vi "example_02_convert.vi"() -> ()   [LabVIEW 2015, in "lv-unit-conversion.lvlib"] (continued)
"is_si_unit"=TRUE, "category"="derived", "base_unit"="m/m3", "conversion_reference"="DERIVED", "is_exact"=TRUE, "a"=0.0, "b"=1000000.0, "c"=1.0, "d"=0.0, "underlying_def"="", "description"=""}, {"symbol"="mi/gal[UK]", "name"="mile per UK gallon", "dimension"="1/L2", "is_si_unit"=TRUE, "category"="derived", "base_unit"="m/m3", "conversion_reference"="DERIVED", "is_exact"=TRUE, "a"=0.0, "b"=1609.344, "c"=0.00454609, "d"=0.0, "underlying_def"="", "description"=""}, {"symbol"="mi/gal[US]", "name"="mile per US gallon", "dimension"="1/L2", "is_si_unit"=TRUE, "category"="derived", "base_unit"="m/m3", "conversion_reference"="DERIVED", "is_exact"=TRUE, "a"=0.0, "b"=1609.344, "c"=0.003785411784, "d"=0.0, "underlying_def"="", "description"=""}, {"symbol"="1/bbl", "name"="per barrel", "dimension"="1/L3", "is_si_unit"=TRUE, "category"="derived", "base_unit"="1/m3", "conversion_reference"="DERIVED", "is_exact"=TRUE, "a"=0.0, "b"=1.0, "c"=0.158987294928, "d"=0.0, "underlying_def"="", "description"=""}, {"symbol"="1/ft3", "name"="per cubic foot", "dimension"="1/L3", "is_si_unit"=TRUE, "category"="derived", "base_unit"="1/m3", "conversion_reference"="DERIVED", "is_exact"=TRUE, "a"=0.0, "b"=1.0, "c"=0.028316846592, "d"=0.0, "underlying_def"="", "description"=""}, {"symbol"="1/gal[UK]", "name"="per UK gallon", "dimension"="1/L3", "is_si_unit"=TRUE, "category"="derived", "base_unit"="1/m3", "conversion_reference"="DERIVED", "is_exact"=TRUE, "a"=0.0, "b"=1.0, "c"=0.00454609, "d"=0.0, "underlying_def"="", "description"=""}, {"symbol"="1/gal[US]", "name"="per US gallon", "dimension"="1/L3", "is_si_unit"=TRUE, "category"="derived", "base_unit"="1/m3", "conversion_reference"="DERIVED", "is_exact"=TRUE, "a"=0.0, "b"=1.0, "c"=0.003785411784, "d"=0.0, "underlying_def"="", "description"=""}, {"symbol"="1/L", "name"="per litre", "dimension"="1/L3", "is_si_unit"=TRUE, "category"="derived", "base_unit"="1/m3", "conversion_reference"="DERIVED", "is_exact"=TRUE, "a"=0.0, "b"=1000.0, "c"=1.0, "d"=0.0, "underlying_def"="", "description"=""}, {"symbol"="1/m3", "name"="per cubic metre", "dimension"="1/L3", "is_si_unit"=TRUE, "category"="derived", "base_unit"="", "conversion_reference"="", "is_exact"=FALSE, "a"=0.0, "b"=0.0, "c"=0.0, "d"=0.0, "underlying_def"="", "description"=""}, {"symbol"="1/g", "name"="per gram", "dimension"="1/M", "is_si_unit"=TRUE, "category"="derived", "base_unit"="1/kg", "conversion_reference"="DERIVED", "is_exact"=TRUE, "a"=0.0, "b"=1000.0, "c"=1.0, "d"=0.0, "underlying_def"="", "description"=""}, {"symbol"="1/lbm", "name"="per pound", "dimension"="1/M", "is_si_unit"=TRUE, "category"="derived", "base_unit"="1/kg", "conversion_reference"="DERIVED", "is_exact"=TRUE, "a"=0.0, "b"=1.0, "c"=0.45359237, "d"=0.0, "underlying_def"="", "description"=""}, {"symbol"="1/kg", "name"="per kilogram", "dimension"="1/M", "is_si_unit"=TRUE, "category"="derived", "base_unit"="", "conversion_reference"="", "is_exact"=FALSE, "a"=0.0, "b"=0.0, "c"=0.0, "d"=0.0, "underlying_def"="", "description"=""}, {"symbol"="1/(kg.s)", "name"="per (kilogram per second)", "dimension"="1/MT", "is_si_unit"=TRUE, "category"="derived", "base_unit"="Bq/kg", "conversion_reference"="DERIVED", "is_exact"=TRUE, "a"=0.0, "b"=1.0, "c"=1.0, "d"=0.0, "underlying_def"="", "description"=""}, {"symbol"="pCi/g", "name"="picocurie per gram", "dimension"="1/MT", "is_si_unit"=TRUE, "category"="derived", "base_unit"="Bq/kg", "conversion_reference"="DERIVED", "is_exact"=TRUE, "a"=0.0, "b"=37.0, "c"=1.0, "d"=0.0, "underlying_def"="", "description"=""}, {"symbol"="Bq/kg", "name"="becquerel per kilogram", "dimension"="1/MT", "is_si_unit"=TRUE, "category"="derived", "base_unit"="", "conversion_reference"="", "is_exact"=FALSE, "a"=0.0, "b"=0.0, "c"=0.0, "d"=0.0, "underlying_def"="1/(kg.s)", "description"=""}, {"symbol"="Ci", "name"="curie", "dimension"="1/T", "is_si_unit"=TRUE, "category"="atom-allowed", "base_unit"="Bq", "conversion_reference"="NIST-SI", "is_exact"=TRUE, "a"=0.0, "b"=37000000000.0, "c"=1.0, "d"=0.0, "underlying_def"="3.7E10 Bq", "description"="The Curie (symbol Ci) is a non-SI unit of radioactivity, named after Marie and Pierre Curie. \n\t\t\t\tIt is defined as 3.7E10 decays per second. \n\t\t\t\tThe SI derived unit of radioactivity is the becquerel (Bq), which equates to one decay per second.\n\t\t\t"}, {"symbol"="Bd", "name"="baud", "dimension"="1/T", "is_si_unit"=TRUE, "category"="atom-allowed", "base_unit"="", "conversion_reference"="", "is_exact"=FALSE, "a"=0.0, "b"=0.0, "c"=0.0, "d"=0.0, "underlying_def"="1/s", "description"="The baud rate is the number of distinct symbols transmitted per second, that is, the number of times \n\t\t\t\tper second the signal carrying the communication varies in strength or frequency. \n\t\t\t\tIf the symbols transmitted have only two states (on or off) then the baud rate is the same as the \n\t\t\t\ttransmission rate in bits per second. \n\t\t\t\t(Adapted from Russ Rowlett's \"A Dictionary of Units of Measurement\" at http://www.unc.edu/~rowlett/units/)\n\t\t\t"}, {"symbol"="Bq", "name"="becquerel", "dimension"="1/T", "is_si_unit"=TRUE, "category"="atom-special", "base_unit"="", "conversion_reference"="", "is_exact"=FALSE, "a"=0.0, "b"=0.0, "c"=0.0, "d"=0.0, "underlying_def"="1/s", "description"="The activity of a radionuclide decaying at the rate of one spontaneous nuclear transition per second"}, {"symbol"="Hz", "name"="hertz", "dimension"="1/T", "is_si_unit"=TRUE, "category"="atom-special", "base_unit"="", "conversion_reference"="", "is_exact"=FALSE, "a"=0.0, "b"=0.0, "c"=0.0, "d"=0.0, "underlying_def"="1/s", "description"="The frequency of a periodic phenomenon of which the period is 1 second."}, {"symbol"="1/a", "name"="per julian-year", "dimension"="1/T", "is_si_unit"=TRUE, "category"="derived", "base_unit"="1/s", "conversion_reference"="DERIVED", "is_exact"=TRUE, "a"=0.0, "b"=1.0, "c"=31557600.0, "d"=0.0, "underlying_def"="", "description"=""}, {"symbol"="1/d", "name"="per day", "dimension"="1/T", "is_si_unit"=TRUE, "category"="derived", "base_unit"="1/s", "conversion_reference"="DERIVED", "is_exact"=TRUE, "a"=0.0, "b"=1.0, "c"=86400.0, "d"=0.0, "underlying_def"="", "description"=""}, {"symbol"="1/h", "name"="per hour", "dimension"="1/T", "is_si_unit"=TRUE, "category"="derived", "base_unit"="1/s", "conversion_reference"="DERIVED", "is_exact"=TRUE, "a"=0.0, "b"=1.0, "c"=3600.0, "d"=0.0, "underlying_def"="", "description"=""}, {"symbol"="1/min", "name"="per minute", "dimension"="1/T", "is_si_unit"=TRUE, "category"="derived", "base_unit"="1/s", "conversion_reference"="DERIVED", "is_exact"=TRUE, "a"=0.0, "b"=1.0, "c"=60.0, "d"=0.0, "underlying_def"="", "description"=""}, {"symbol"="1/ms", "name"="per millisecond", "dimension"="1/T", "is_si_unit"=TRUE, "category"="derived", "base_unit"="1/s", "conversion_reference"="DERIVED", "is_exact"=TRUE, "a"=0.0, "b"=1000.0, "c"=1.0, "d"=0.0, "underlying_def"="", "description"=""}, {"symbol"="1/us", "name"="per microsecond", "dimension"="1/T", "is_si_unit"=TRUE, "category"="derived", "base_unit"="1/s", "conversion_reference"="DERIVED", "is_exact"=TRUE, "a"=0.0, "b"=1000000.0, "c"=1.0, "d"=0.0, "underlying_def"="", "description"=""}, {"symbol"="1/wk", "name"="per week", "dimension"="1/T", "is_si_unit"=TRUE, "category"="derived", "base_unit"="1/s", "conversion_reference"="DERIVED", "is_exact"=TRUE, "a"=0.0, "b"=1.0, "c"=604800.0, "d"=0.0, "underlying_def"="", "description"=""}, {"symbol"="byte/s", "name"="byte per second", "dimension"="1/T", "is_si_unit"=TRUE, "category"="derived", "base_unit"="bit/s", "conversion_reference"="DERIVED", "is_exact"=TRUE, "a"=0.0, "b"=8.0, "c"=1.0, "d"=0.0, "underlying_def"="", "description"=""}, {"symbol"="1/s", "name"="per second", "dimension"="1/T", "is_si_unit"=TRUE, "category"="derived", "base_unit"="", "conversion_reference"="", "is_exact"=FALSE, "a"=0.0, "b"=0.0, "c"=0.0, "d"=0.0, "underlying_def"="", "description"=""}, {"symbol"="bit/s", "name"="bit per second", "dimension"="1/T", "is_si_unit"=TRUE, "category"="derived", "base_unit"="", "conversion_reference"="", "is_exact"=FALSE, "a"=0.0, "b"=0.0, "c"=0.0, "d"=0.0, "underlying_def"="1/s", "description"="A unit of transmission speed, equal to one bit per second."}, {"symbol"="m3/(s.m3)", "name"="cubic metre per time cubic metre", "dimension"="1/T", "is_si_unit"=TRUE, "category"="derived", "base_unit"="", "conversion_reference"="", "is_exact"=FALSE, "a"=0.0, "b"=0.0, "c"=0.0, "d"=0.0, "underlying_def"="1/s", "description"=""}, {"symbol"="bbl/(d.acre.ft)", "name"="barrel per day acre foot", "dimension"="1/T", "is_si_unit"=TRUE, "category"="derived", "base_unit"="m3/(s.m3)", "conversion_reference"="DERIVED", "is_exact"=TRUE, "a"=0.0, "b"=2464298.1427778574, "c"=1651882180608000.0, "d"=0.0, "underlying_def"="", "description"=""}, {"symbol"="GBq", "name"="gigabecquerel", "dimension"="1/T", "is_si_unit"=TRUE, "category"="prefixed", "base_unit"="Bq", "conversion_reference"="DERIVED", "is_exact"=TRUE, "a"=0.0, "b"=1000000000.0, "c"=1.0, "d"=0.0, "underlying_def"="", "description"=""}, {"symbol"="MBq", "name"="megabecquerel", "dimension"="1/T", "is_si_unit"=TRUE, "category"="prefixed", "base_unit"="Bq", "conversion_reference"="DERIVED", "is_exact"=TRUE, "a"=0.0, "b"=1000000.0, "c"=1.0, "d"=0.0, "underlying_def"="", "description"=""}, {"symbol"="mCi", "name"="thousandth of curie", "dimension"="1/T", "is_si_unit"=TRUE, "category"="prefixed", "base_unit"="Bq", "conversion_reference"="DERIVED", "is_exact"=TRUE, "a"=0.0, "b"=37000000.0, "c"=1.0, "d"=0.0, "underlying_def"="", "description"=""}, {"symbol"="nCi", "name"="nanocurie", "dimension"="1/T", "is_si_unit"=TRUE, "category"="prefixed", "base_unit"="Bq", "conversion_reference"="DERIVED", "is_exact"=TRUE, "a"=0.0, "b"=37.0, "c"=1.0, "d"=0.0, "underlying_def"="", "description"=""}, {"symbol"="pCi", "name"="picocurie", "dimension"="1/T", "is_si_unit"=TRUE, "category"="prefixed", "base_unit"="Bq", "conversion_reference"="DERIVED", "is_exact"=TRUE, "a"=0.0, "b"=0.037, "c"=1.0, "d"=0.0, "underlying_def"="", "description"=""}, {"symbol"="TBq", "name"="terabecquerel", "dimension"="1/T", "is_si_unit"=TRUE, "category"="prefixed", "base_unit"="Bq", "conversion_reference"="DERIVED", "is_exact"=TRUE, "a"=0.0, "b"=1000000000000.0, "c"=1.0, "d"=0.0, "underlying_def"="", "description"=""}, {"symbol"="uCi", "name"="millionth of curie", "dimension"="1/T", "is_si_unit"=TRUE, "category"="prefixed", "base_unit"="Bq", "conversion_reference"="DERIVED", "is_exact"=TRUE, "a"=0.0, "b"=37000.0, "c"=1.0, "d"=0.0, "underlying_def"="", "description"=""}, {"symbol"="cHz", "name"="centihertz", "dimension"="1/T", "is_si_unit"=TRUE, "category"="prefixed", "base_unit"="Hz", "conversion_reference"="DERIVED", "is_exact"=TRUE, "a"=0.0, "b"=0.01, "c"=1.0, "d"=0.0, "underlying_def"="", "description"=""}, {"symbol"="dHz", "name"="decihertz", "dimension"="1/T", "is_si_unit"=TRUE, "category"="prefixed", "base_unit"="Hz", "conversion_reference"="DERIVED", "is_exact"=TRUE, "a"=0.0, "b"=0.1, "c"=1.0, "d"=0.0, "underlying_def"="", "description"=""}, {"symbol"="EHz", "name"="exahertz", "dimension"="1/T", "is_si_unit"=TRUE, "category"="prefixed", "base_unit"="Hz", "conversion_reference"="DERIVED", "is_exact"=TRUE, "a"=0.0, "b"=1e+18, "c"=1.0, "d"=0.0, "underlying_def"="", "description"=""}, {"symbol"="fHz", "name"="femtohertz", "dimension"="1/T", "is_si_unit"=TRUE, "category"="prefixed", "base_unit"="Hz", "conversion_reference"="DERIVED", "is_exact"=TRUE, "a"=0.0, "b"=1e-15, "c"=1.0, "d"=0.0, "underlying_def"="", "description"=""}, {"symbol"="GHz", "name"="gigahertz", "dimension"="1/T", "is_si_unit"=TRUE, "category"="prefixed", "base_unit"="Hz", "conversion_reference"="DERIVED", "is_exact"=TRUE, "a"=0.0, "b"=1000000000.0, "c"=1.0, "d"=0.0, "underlying_def"="", "description"=""}, {"symbol"="kHz", "name"="kilohertz", "dimension"="1/T", "is_si_unit"=TRUE, "category"="prefixed", "base_unit"="Hz", "conversion_reference"="DERIVED", "is_exact"=TRUE, "a"=0.0, "b"=1000.0, "c"=1.0, "d"=0.0, "underlying_def"="", "description"=""}, {"symbol"="mHz", "name"="millihertz", "dimension"="1/T", "is_si_unit"=TRUE, "category"="prefixed", "base_unit"="Hz", "conversion_reference"="DERIVED", "is_exact"=TRUE, "a"=0.0, "b"=0.001, "c"=1.0, "d"=0.0, "underlying_def"="", "description"=""}, {"symbol"="MHz", "name"="megahertz", "dimension"="1/T", "is_si_unit"=TRUE, "category"="prefixed", "base_unit"="Hz", "conversion_reference"="DERIVED", "is_exact"=TRUE, "a"=0.0, "b"=1000000.0, "c"=1.0, "d"=0.0, "underlying_def"="", "description"=""}, {"symbol"="nHz", "name"="nanohertz", "dimension"="1/T", "is_si_unit"=TRUE, "category"="prefixed", "base_unit"="Hz", "conversion_reference"="DERIVED", "is_exact"=TRUE, "a"=0.0, "b"=1e-09, "c"=1.0, "d"=0.0, "underlying_def"="", "description"=""}, {"symbol"="pHz", "name"="picohertz", "dimension"="1/T", "is_si_unit"=TRUE, "category"="prefixed", "base_unit"="Hz", "conversion_reference"="DERIVED", "is_exact"=TRUE, "a"=0.0, "b"=1e-12, "c"=1.0, "d"=0.0, "underlying_def"="", "description"=""}, {"symbol"="THz", "name"="terahertz", "dimension"="1/T", "is_si_unit"=TRUE, "category"="prefixed", "base_unit"="Hz", "conversion_reference"="DERIVED", "is_exact"=TRUE, "a"=0.0, "b"=1000000000000.0, "c"=1.0, "d"=0.0, "underlying_def"="", "description"=""}, {"symbol"="uHz", "name"="microhertz", "dimension"="1/T", "is_si_unit"=TRUE, "category"="prefixed", "base_unit"="Hz", "conversion_reference"="DERIVED", "is_exact"=TRUE, "a"=0.0, "b"=1e-06, "c"=1.0, "d"=0.0, "underlying_def"="", "description"=""}, {"symbol"="rad", "name"="radian", "dimension"="A", "is_si_unit"=TRUE, "category"="atom-special", "base_unit"="", "conversion_reference"="", "is_exact"=FALSE, "a"=0.0, "b"=0.0, "c"=0.0, "d"=0.0, "underlying_def"="", "description"="The radian is the plane angle between two radii of a circle that cut of, on the circumference,an arc \n\t\t\t\tequal in length to the radius.\n\t\t\t"}, {"symbol"="ccgr", "name"="centesimal-second", "dimension"="A", "is_si_unit"=TRUE, "category"="atom", "base_unit"="rad", "conversion_reference"="EPSG", "is_exact"=TRUE, "a"=0.0, "b"=0.0, "c"=2000000.0, "d"=0.0, "underlying_def"="1/100 cgr", "description"="One hundredth of a centesimal-minute."}, {"symbol"="cgr", "name"="centesimal-minute", "dimension"="A", "is_si_unit"=TRUE, "category"="atom", "base_unit"="rad", "conversion_reference"="EPSG", "is_exact"=TRUE, "a"=0.0, "b"=0.0, "c"=20000.0, "d"=0.0, "underlying_def"="1/100 gon", "description"="One hundredth of a centesimal degree (also known as grad, grade or gon)"}, {"symbol"="dega", "name"="angular degree", "dimension"="A", "is_si_unit"=TRUE, "category"="atom-allowed", "base_unit"="rad", "conversion_reference"="NIST-SI", "is_exact"=TRUE, "a"=0.0, "b"=0.0, "c"=180.0, "d"=0.0, "underlying_def"="", "description"="1/360 of a full circle = PI /180 radians"}, {"symbol"="gon", "name"="gon", "dimension"="A", "is_si_unit"=TRUE, "category"="atom", "base_unit"="rad", "conversion_reference"="EPSG", "is_exact"=TRUE, "a"=0.0, "b"=0.0, "c"=200.0, "d"=0.0, "underlying_def"="360/400 dega", "description"="1/400 of a turn (full circle). Also known as gradian, grad, or grade."}, {"symbol"="mila", "name"="angular mil", "dimension"="A", "is_si_unit"=TRUE, "category"="atom", "base_unit"="rad", "conversion_reference"="EPSG", "is_exact"=TRUE, "a"=0.0, "b"=0.0, "c"=3200.0, "d"=0.0, "underlying_def"="360/6400 dega", "description"="Angle subtended by 1/6400 part of a circle."}, {"symbol"="mina", "name"="angular minute", "dimension"="A", "is_si_unit"=TRUE, "category"="atom-allowed", "base_unit"="rad", "conversion_reference"="NIST-SI", "is_exact"=TRUE, "a"=0.0, "b"=0.0, "c"=10800.0, "d"=0.0, "underlying_def"="1/60 dega", "description"="1/60 of an angular degree. ((pi/180) / 60) radians"}, {"symbol"="rev", "name"="revolution", "dimension"="A", "is_si_unit"=TRUE, "category"="atom", "base_unit"="rad", "conversion_reference"="DEFINITION", "is_exact"=TRUE, "a"=0.0, "b"=2.0, "c"=1.0, "d"=0.0, "underlying_def"="360 dega", "description"="One complete 360 degree rotational cycle."}, {"symbol"="seca", "name"="angular second", "dimension"="A", "is_si_unit"=TRUE, "category"="atom-allowed", "base_unit"="rad", "conversion_reference"="NIST-SI", "is_exact"=TRUE, "a"=0.0, "b"=0.0, "c"=648000.0, "d"=0.0, "underlying_def"="1/60 mina", "description"="1/60 of an angular minute. ((pi/180) / 3600) radians"}, {"symbol"="0.001 seca", "name"="angular millisecond", "dimension"="A", "is_si_unit"=TRUE, "category"="derived", "base_unit"="rad", "conversion_reference"="DERIVED", "is_exact"=TRUE, "a"=0.0, "b"=0.0, "c"=648000000.0, "d"=0.0, "underlying_def"="", "description"=""}, {"symbol"="krad", "name"="kiloradian", "dimension"="A", "is_si_unit"=TRUE, "category"="prefixed", "base_unit"="rad", "conversion_reference"="DERIVED", "is_exact"=TRUE, "a"=0.0, "b"=1000.0, "c"=1.0, "d"=0.0, "underlying_def"="", "description"=""}, {"symbol"="mrad", "name"="milliradian", "dimension"="A", "is_si_unit"=TRUE, "category"="prefixed", "base_unit"="rad", "conversion_reference"="DERIVED", "is_exact"=TRUE, "a"=0.0, "b"=0.001, "c"=1.0, "d"=0.0, "underlying_def"="", "description"=""}, {"symbol"="Mrad", "name"="megaradian", "dimension"="A", "is_si_unit"=TRUE, "category"="prefixed", "base_unit"="rad", "conversion_reference"="DERIVED", "is_exact"=TRUE, "a"=0.0, "b"=1000000.0, "c"=1.0, "d"=0.0, "underlying_def"="", "description"=""}, {"symbol"="urad", "name"="microradian", "dimension"="A", "is_si_unit"=TRUE, "category"="prefixed", "base_unit"="rad", "conversion_reference"="DERIVED", "is_exact"=TRUE, "a"=0.0, "b"=1e-06, "c"=1.0, "d"=0.0, "underlying_def"="", "description"=""}, {"symbol"="rad/m", "name"="radian per metre", "dimension"="A/L", "is_si_unit"=TRUE, "category"="derived", "base_unit"="", "conversion_reference"="", "is_exact"=FALSE, "a"=0.0, "b"=0.0, "c"=0.0, "d"=0.0, "underlying_def"="", "description"=""}, {"symbol"="0.01 dega/ft", "name"="angular degree per hundred foot", "dimension"="A/L", "is_si_unit"=TRUE, "category"="derived", "base_unit"="rad/m", "conversion_reference"="DERIVED", "is_exact"=TRUE, "a"=0.0, "b"=0.0, "c"=5486.4, "d"=0.0, "underlying_def"="", "description"=""}, {"symbol"="1/30 dega/ft", "name"="angular degree per thirty foot", "dimension"="A/L", "is_si_unit"=TRUE, "category"="derived", "base_unit"="rad/m", "conversion_reference"="DERIVED", "is_exact"=TRUE, "a"=0.0, "b"=0.0, "c"=1645.92, "d"=0.0, "underlying_def"="", "description"=""}, {"symbol"="1/30 dega/m", "name"="angular degree per thirty metre", "dimension"="A/L", "is_si_unit"=TRUE, "category"="derived", "base_unit"="rad/m", "conversion_reference"="DERIVED", "is_exact"=TRUE, "a"=0.0, "b"=0.0, "c"=5400.0, "d"=0.0, "underlying_def"="", "description"="((pi/180) / 30) radian per metre"}, {"symbol"="dega/ft", "name"="angular degree per foot", "dimension"="A/L", "is_si_unit"=TRUE, "category"="derived", "base_unit"="rad/m", "conversion_reference"="DERIVED", "is_exact"=TRUE, "a"=0.0, "b"=0.0, "c"=54.864, "d"=0.0, "underlying_def"="", "description"=""}, {"symbol"="dega/m", "name"="angular degree per metre", "dimension"="A/L", "is_si_unit"=TRUE, "category"="derived", "base_unit"="rad/m", "conversion_reference"="DERIVED", "is_exact"=TRUE, "a"=0.0, "b"=0.0, "c"=180.0, "d"=0.0, "underlying_def"="", "description"=""}, {"symbol"="rad/ft", "name"="radian per foot", "dimension"="A/L", "is_si_unit"=TRUE, "category"="derived", "base_unit"="rad/m", "conversion_reference"="DERIVED", "is_exact"=TRUE, "a"=0.0, "b"=1.0, "c"=0.3048, "d"=0.0, "underlying_def"="", "description"=""}, {"symbol"="rev/ft", "name"="revolution per foot", "dimension"="A/L", "is_si_unit"=TRUE, "category"="derived", "base_unit"="rad/m", "conversion_reference"="DERIVED", "is_exact"=TRUE, "a"=0.0, "b"=2.0, "c"=0.3048, "d"=0.0, "underlying_def"="", "description"=""}, {"symbol"="rev/m", "name"="revolution per metre", "dimension"="A/L", "is_si_unit"=TRUE, "category"="derived", "base_unit"="rad/m", "conversion_reference"="DERIVED", "is_exact"=TRUE, "a"=0.0, "b"=2.0, "c"=1.0, "d"=0.0, "underlying_def"="", "description"=""}, {"symbol"="rad/m3", "name"="radian per cubic metre", "dimension"="A/L3", "is_si_unit"=TRUE, "category"="derived", "base_unit"="", "conversion_reference"="", "is_exact"=FALSE, "a"=0.0, "b"=0.0, "c"=0.0, "d"=0.0, "underlying_def"="", "description"=""}, {"symbol"="rad/ft3", "name"="radian per cubic foot", "dimension"="A/L3", "is_si_unit"=TRUE, "category"="derived", "base_unit"="rad/m3", "conversion_reference"="DERIVED", "is_exact"=TRUE, "a"=0.0, "b"=1.0, "c"=0.028316846592, "d"=0.0, "underlying_def"="", "description"=""}, {"symbol"="rpm", "name"="revolution per minute", "dimension"="A/T", "is_si_unit"=TRUE, "category"="atom", "base_unit"="rad/s", "conversion_reference"="DERIVED", "is_exact"=TRUE, "a"=0.0, "b"=2.0, "c"=60.0, "d"=0.0, "underlying_def"="rev/min", "description"=""}, {"symbol"="rad/s", "name"="radian per second", "dimension"="A/T", "is_si_unit"=TRUE, "category"="derived", "base_unit"="", "conversion_reference"="", "is_exact"=FALSE, "a"=0.0, "b"=0.0, "c"=0.0, "d"=0.0, "underlying_def"="", "description"=""}, {"symbol"="dega/h", "name"="angular degree per hour", "dimension"="A/T", "is_si_unit"=TRUE, "category"="derived", "base_unit"="rad/s", "conversion_reference"="DERIVED", "is_exact"=TRUE, "a"=0.0, "b"=0.0, "c"=648000.0, "d"=0.0, "underlying_def"="", "description"="((pi/180) / 3600) radian per second"}, {"symbol"="dega/min", "name"="angular degree per minute", "dimension"="A/T", "is_si_unit"=TRUE, "category"="derived", "base_unit"="rad/s", "conversion_reference"="DERIVED", "is_exact"=TRUE, "a"=0.0, "b"=0.0, "c"=10800.0, "d"=0.0, "underlying_def"="", "description"="((pi/180) / 60) radian per second"}, {"symbol"="dega/s", "name"="angular degree per second", "dimension"="A/T", "is_si_unit"=TRUE, "category"="derived", "base_unit"="rad/s", "conversion_reference"="DERIVED", "is_exact"=TRUE, "a"=0.0, "b"=0.0, "c"=180.0, "d"=0.0, "underlying_def"="", "description"="(pi/180) radian per second"}, {"symbol"="rev/s", "name"="revolution per second", "dimension"="A/T", "is_si_unit"=TRUE, "category"="derived", "base_unit"="rad/s", "conversion_reference"="DERIVED", "is_exact"=TRUE, "a"=0.0, "b"=2.0, "c"=1.0, "d"=0.0, "underlying_def"="", "description"=""}, {"symbol"="rad/s2", "name"="radian per second squared", "dimension"="A/T2", "is_si_unit"=TRUE, "category"="derived", "base_unit"="", "conversion_reference"="", "is_exact"=FALSE, "a"=0.0, "b"=0.0, "c"=0.0, "d"=0.0, "underlying_def"="", "description"=""}, {"symbol"="rpm/s", "name"="(revolution per minute) per second", "dimension"="A/T2", "is_si_unit"=TRUE, "category"="derived", "base_unit"="rad/s2", "conversion_reference"="DERIVED", "is_exact"=TRUE, "a"=0.0, "b"=2.0, "c"=60.0, "d"=0.0, "underlying_def"="", "description"=""}, {"symbol"="deltaC", "name"="delta Celsius", "dimension"="D", "is_si_unit"=TRUE, "category"="atom-special", "base_unit"="deltaK", "conversion_reference"="NIST-SI", "is_exact"=TRUE, "a"=0.0, "b"=1.0, "c"=1.0, "d"=0.0, "underlying_def"="deltaK", "description"="Change in degree Celsius. \n\t\t\t\tThe degree Celsius and the kelvin are equal in size, so that the numerical value of a temperature \n\t\t\t\tdifference or temperature interval is the same when expressed in either degrees Celsius or in \n\t\t\t\tkelvins (because the offset cancels). \n\t\t\t\tFor temperature intervals rather than specific temperatures, 1 deltaF = 1 deltaR = 5/9 deltaC = 5/9 deltaK.\n\t\t\t"}, {"symbol"="deltaF", "name"="delta Fahrenheit", "dimension"="D", "is_si_unit"=TRUE, "category"="atom", "base_unit"="deltaK", "conversion_reference"="NIST-SI", "is_exact"=TRUE, "a"=0.0, "b"=5.0, "c"=9.0, "d"=0.0, "underlying_def"="", "description"="Change in degrees Fahrenheit. \n\t\t\t\tKelvin=(Fahrenheit + 459.67) x 5/9 so a difference in Fahrenheit temperature cancels out the 459.67 \n\t\t\t\toffset. \n\t\t\t\tFor temperature intervals rather than specific temperatures, 1 deltaF = 1 deltaR = 5/9 deltaC = 5/9 deltaK.\n\t\t\t"}, {"symbol"="deltaR", "name"="delta Rankine", "dimension"="D", "is_si_unit"=TRUE, "category"="atom", "base_unit"="deltaK", "conversion_reference"="NIST-SI", "is_exact"=TRUE, "a"=0.0, "b"=5.0, "c"=9.0, "d"=0.0, "underlying_def"="", "description"="Change in degrees Rankine. \n\t\t\t\tRankine = (Celsius + 273.15) x 9/5 so a difference in Fahrenheit temperature cancels out the 273.15 \n\t\t\t\toffset. \n\t\t\t\tFor temperature intervals rather than specific temperatures, 1 deltaF = 1 deltaR = 5/9 deltaC = 5/9 deltaK.\n\t\t\t"}, {"symbol"="deltaK", "name"="delta kelvin", "dimension"="D", "is_si_unit"=TRUE, "category"="atom-special", "base_unit"="", "conversion_reference"="", "is_exact"=FALSE, "a"=0.0, "b"=0.0, "c"=0.0, "d"=0.0, "underlying_def"="", "description"="Change in kelvin. \n\t\t\t\tA zero difference in Kelvin temperature is not the same as being at zero on the Kelvin temperature \n\t\t\t\tscale. \n\t\t\t\tThe degree Celsius and the kelvin are equal in size, so that the numerical value of a temperature \n\t\t\t\tdifference or temperature interval is the same when expressed in either degrees Celsius or in kelvins.\n\t\t\t"}, {"symbol"="0.01 deltaF/ft", "name"="delta Fahrenheit per hundred foot", "dimension"="D/L", "is_si_unit"=TRUE, "category"="derived", "base_unit"="deltaK/m", "conversion_reference"="DERIVED", "is_exact"=TRUE, "a"=0.0, "b"=5.0, "c"=274.32, "d"=0.0, "underlying_def"="", "description"=""}, {"symbol"="deltaC/ft", "name"="delta Celsius per foot", "dimension"="D/L", "is_si_unit"=TRUE, "category"="derived", "base_unit"="deltaK/m", "conversion_reference"="DERIVED", "is_exact"=TRUE, "a"=0.0, "b"=1.0, "c"=0.3048, "d"=0.0, "underlying_def"="", "description"=""}, {"symbol"="deltaC/hm", "name"="delta Celsius per hectometre", "dimension"="D/L", "is_si_unit"=TRUE, "category"="derived", "base_unit"="deltaK/m", "conversion_reference"="DERIVED", "is_exact"=TRUE, "a"=0.0, "b"=0.01, "c"=1.0, "d"=0.0, "underlying_def"="", "description"=""}, {"symbol"="deltaC/km", "name"="delta Celsius per kilometre", "dimension"="D/L", "is_si_unit"=TRUE, "category"="derived", "base_unit"="deltaK/m", "conversion_reference"="DERIVED", "is_exact"=TRUE, "a"=0.0, "b"=0.001, "c"=1.0, "d"=0.0, "underlying_def"="", "description"=""}, {"symbol"="deltaC/m", "name"="delta Celsius per metre", "dimension"="D/L", "is_si_unit"=TRUE, "category"="derived", "base_unit"="deltaK/m", "conversion_reference"="DERIVED", "is_exact"=TRUE, "a"=0.0, "b"=1.0, "c"=1.0, "d"=0.0, "underlying_def"="", "description"=""}, {"symbol"="deltaF/ft", "name"="delta Fahrenheit per foot", "dimension"="D/L", "is_si_unit"=TRUE, "category"="derived", "base_unit"="deltaK/m", "conversion_reference"="DERIVED", "is_exact"=TRUE, "a"=0.0, "b"=5.0, "c"=2.7432, "d"=0.0, "underlying_def"="", "description"=""}, {"symbol"="deltaF/m", "name"="delta Fahrenheit per metre", "dimension"="D/L", "is_si_unit"=TRUE, "category"="derived", "base_unit"="deltaK/m", "conversion_reference"="DERIVED", "is_exact"=TRUE, "a"=0.0, "b"=5.0, "c"=9.0, "d"=0.0, "underlying_def"="", "description"=""}, {"symbol"="deltaK/km", "name"="delta kelvin per kilometre", "dimension"="D/L", "is_si_unit"=TRUE, "category"="derived", "base_unit"="deltaK/m", "conversion_reference"="DERIVED", "is_exact"=TRUE, "a"=0.0, "b"=0.001, "c"=1.0, "d"=0.0, "underlying_def"="", "description"=""}, {"symbol"="deltaK/m", "name"="delta kelvin per metre", "dimension"="D/L", "is_si_unit"=TRUE, "category"="derived", "base_unit"="", "conversion_reference"="", "is_exact"=FALSE, "a"=0.0, "b"=0.0, "c"=0.0, "d"=0.0, "underlying_def"="", "description"=""}, {"symbol"="deltaC/h", "name"="delta Celsius per hour", "dimension"="D/T", "is_si_unit"=TRUE, "category"="derived", "base_unit"="deltaK/s", "conversion_reference"="DERIVED", "is_exact"=TRUE, "a"=0.0, "b"=1.0, "c"=3600.0, "d"=0.0, "underlying_def"="", "description"=""}, {"symbol"="deltaC/min", "name"="delta Celsius per minute", "dimension"="D/T", "is_si_unit"=TRUE, "category"="derived", "base_unit"="deltaK/s", "conversion_reference"="DERIVED", "is_exact"=TRUE, "a"=0.0, "b"=1.0, "c"=60.0, "d"=0.0, "underlying_def"="", "description"=""}, {"symbol"="deltaC/s", "name"="delta Celsius per second", "dimension"="D/T", "is_si_unit"=TRUE, "category"="derived", "base_unit"="deltaK/s", "conversion_reference"="DERIVED", "is_exact"=TRUE, "a"=0.0, "b"=1.0, "c"=1.0, "d"=0.0, "underlying_def"="", "description"=""}, {"symbol"="deltaF/h", "name"="delta Fahrenheit per hour", "dimension"="D/T", "is_si_unit"=TRUE, "category"="derived", "base_unit"="deltaK/s", "conversion_reference"="DERIVED", "is_exact"=TRUE, "a"=0.0, "b"=5.0, "c"=32400.0, "d"=0.0, "underlying_def"="", "description"=""}, {"symbol"="deltaF/min", "name"="delta Fahrenheit per minute", "dimension"="D/T", "is_si_unit"=TRUE, "category"="derived", "base_unit"="deltaK/s", "conversion_reference"="DERIVED", "is_exact"=TRUE, "a"=0.0, "b"=5.0, "c"=540.0, "d"=0.0, "underlying_def"="", "description"=""}, {"symbol"="deltaF/s", "name"="delta Fahrenheit per second", "dimension"="D/T", "is_si_unit"=TRUE, "category"="derived", "base_unit"="deltaK/s", "conversion_reference"="DERIVED", "is_exact"=TRUE, "a"=0.0, "b"=5.0, "c"=9.0, "d"=0.0, "underlying_def"="", "description"=""}, {"symbol"="deltaK/s", "name"="delta kelvin per second", "dimension"="D/T", "is_si_unit"=TRUE, "category"="derived", "base_unit"="", "conversion_reference"="", "is_exact"=FALSE, "a"=0.0, "b"=0.0, "c"=0.0, "d"=0.0, "underlying_def"="", "description"=""}, {"symbol"="deltaC/kPa", "name"="delta Celsius per kilopascal", "dimension"="DLT2/M", "is_si_unit"=TRUE, "category"="derived", "base_unit"="deltaK/Pa", "conversion_reference"="DERIVED", "is_exact"=TRUE, "a"=0.0, "b"=0.001, "c"=1.0, "d"=0.0, "underlying_def"="", "description"=""}, {"symbol"="deltaF/psi", "name"="delta Fahrenheit per psi", "dimension"="DLT2/M", "is_si_unit"=TRUE, "category"="derived", "base_unit"="deltaK/Pa", "conversion_reference"="DERIVED", "is_exact"=TRUE, "a"=0.0, "b"=0.0032258, "c"=40.0339945373445, "d"=0.0, "underlying_def"="", "description"=""}, {"symbol"="deltaK/Pa", "name"="delta kelvin per Pascal", "dimension"="DLT2/M", "is_si_unit"=TRUE, "category"="derived", "base_unit"="", "conversion_reference"="", "is_exact"=FALSE, "a"=0.0, "b"=0.0, "c"=0.0, "d"=0.0, "underlying_def"="", "description"=""}, {"symbol"="deltaK/W", "name"="delta kelvin per watt", "dimension"="DT3/L2M", "is_si_unit"=TRUE, "category"="derived", "base_unit"="", "conversion_reference"="", "is_exact"=FALSE, "a"=0.0, "b"=0.0, "c"=0.0, "d"=0.0, "underlying_def"="", "description"=""}, {"symbol"="deltaC.m2.h/kcal[th]", "name"="delta Celsius square metre hour per thousand calory", "dimension"="DT3/M", "is_si_unit"=TRUE, "category"="derived", "base_unit"="deltaK.m2/W", "conversion_reference"="DERIVED", "is_exact"=TRUE, "a"=0.0, "b"=3600.0, "c"=4184.0, "d"=0.0, "underlying_def"="", "description"=""}, {"symbol"="deltaF.ft2.h/Btu[IT]", "name"="delta Fahrenheit square foot hour per BTU", "dimension"="DT3/M", "is_si_unit"=TRUE, "category"="derived", "base_unit"="deltaK.m2/W", "conversion_reference"="DERIVED", "is_exact"=TRUE, "a"=0.0, "b"=1672.25472, "c"=9495.50267358, "d"=0.0, "underlying_def"="", "description"=""}, {"symbol"="deltaK.m2/kW", "name"="delta kelvin square metre per kilowatt", "dimension"="DT3/M", "is_si_unit"=TRUE, "category"="derived", "base_unit"="deltaK.m2/W", "conversion_reference"="DERIVED", "is_exact"=TRUE, "a"=0.0, "b"=0.001, "c"=1.0, "d"=0.0, "underlying_def"="", "description"=""}, {"symbol"="deltaK.m2/W", "name"="delta kelvin square metre per watt", "dimension"="DT3/M", "is_si_unit"=TRUE, "category"="derived", "base_unit"="", "conversion_reference"="", "is_exact"=FALSE, "a"=0.0, "b"=0.0, "c"=0.0, "d"=0.0, "underlying_def"="", "description"=""}, {"symbol"="A", "name"="ampere", "dimension"="I", "is_si_unit"=TRUE, "category"="atom-base", "base_unit"="", "conversion_reference"="", "is_exact"=FALSE, "a"=0.0, "b"=0.0, "c"=0.0, "d"=0.0, "underlying_def"="", "description"="The ampere is that constant current which, if maintained in two straight parallel conductors of \n\t\t\t\tinfinite length, of negligible circular cross section, and placed 1 metre apart in vacuum, would \n\t\t\t\tproduce between these conductors a force equal to 2 x 10**-7 newton per metre of length.\n\t\t\t"}, {"symbol"="cA", "name"="centiampere", "dimension"="I", "is_si_unit"=TRUE, "category"="prefixed", "base_unit"="A", "conversion_reference"="DERIVED", "is_exact"=TRUE, "a"=0.0, "b"=0.01, "c"=1.0, "d"=0.0, "underlying_def"="", "description"=""}, {"symbol"="dA", "name"="deciampere", "dimension"="I", "is_si_unit"=TRUE, "category"="prefixed", "base_unit"="A", "conversion_reference"="DERIVED", "is_exact"=TRUE, "a"=0.0, "b"=0.1, "c"=1.0, "d"=0.0, "underlying_def"="", "description"=""}, {"symbol"="EA", "name"="exaampere", "dimension"="I", "is_si_unit"=TRUE, "category"="prefixed", "base_unit"="A", "conversion_reference"="DERIVED", "is_exact"=TRUE, "a"=0.0, "b"=1e+18, "c"=1.0, "d"=0.0, "underlying_def"="", "description"=""}, {"symbol"="fA", "name"="femtoampere", "dimension"="I", "is_si_unit"=TRUE, "category"="prefixed", "base_unit"="A", "conversion_reference"="DERIVED", "is_exact"=TRUE, "a"=0.0, "b"=1e-15, "c"=1.0, "d"=0.0, "underlying_def"="", "description"=""}, {"symbol"="GA", "name"="gigaampere", "dimension"="I", "is_si_unit"=TRUE, "category"="prefixed", "base_unit"="A", "conversion_reference"="DERIVED", "is_exact"=TRUE, "a"=0.0, "b"=1000000000.0, "c"=1.0, "d"=0.0, "underlying_def"="", "description"=""}, {"symbol"="kA", "name"="kiloampere", "dimension"="I", "is_si_unit"=TRUE, "category"="prefixed", "base_unit"="A", "conversion_reference"="DERIVED", "is_exact"=TRUE, "a"=0.0, "b"=1000.0, "c"=1.0, "d"=0.0, "underlying_def"="", "description"=""}, {"symbol"="mA", "name"="milliampere", "dimension"="I", "is_si_unit"=TRUE, "category"="prefixed", "base_unit"="A", "conversion_reference"="DERIVED", "is_exact"=TRUE, "a"=0.0, "b"=0.001, "c"=1.0, "d"=0.0, "underlying_def"="", "description"=""}, {"symbol"="MA", "name"="megaampere", "dimension"="I", "is_si_unit"=TRUE, "category"="prefixed", "base_unit"="A", "conversion_reference"="DERIVED", "is_exact"=TRUE, "a"=0.0, "b"=1000000.0, "c"=1.0, "d"=0.0, "underlying_def"="", "description"=""}, {"symbol"="nA", "name"="nanoampere", "dimension"="I", "is_si_unit"=TRUE, "category"="prefixed", "base_unit"="A", "conversion_reference"="DERIVED", "is_exact"=TRUE, "a"=0.0, "b"=1e-09, "c"=1.0, "d"=0.0, "underlying_def"="", "description"=""}, {"symbol"="pA", "name"="picoampere", "dimension"="I", "is_si_unit"=TRUE, "category"="prefixed", "base_unit"="A", "conversion_reference"="DERIVED", "is_exact"=TRUE, "a"=0.0, "b"=1e-12, "c"=1.0, "d"=0.0, "underlying_def"="", "description"=""}, {"symbol"="TA", "name"="teraampere", "dimension"="I", "is_si_unit"=TRUE, "category"="prefixed", "base_unit"="A", "conversion_reference"="DERIVED", "is_exact"=TRUE, "a"=0.0, "b"=1000000000000.0, "c"=1.0, "d"=0.0, "underlying_def"="", "description"=""}, {"symbol"="uA", "name"="microampere", "dimension"="I", "is_si_unit"=TRUE, "category"="prefixed", "base_unit"="A", "conversion_reference"="DERIVED", "is_exact"=TRUE, "a"=0.0, "b"=1e-06, "c"=1.0, "d"=0.0, "underlying_def"="", "description"=""}, {"symbol"="Oe", "name"="oersted", "dimension"="I/L", "is_si_unit"=TRUE, "category"="atom", "base_unit"="A/m", "conversion_reference"="NIST-SI", "is_exact"=TRUE, "a"=0.0, "b"=1000.0, "c"=4.0, "d"=0.0, "underlying_def"="", "description"="1 Oe corresponds to (1000/(4*pi)) A/m. \n\t\t\t\tThis unit is part of the so-called electromagnetic three-dimensional CGS system and cannot strictly \n\t\t\t\tspeaking be compared to the corresponding SI unit, which has four dimensions when only mechanical \n\t\t\t\tand electric quantities are considered.\n\t\t\t"}, {"symbol"="A/mm", "name"="ampere per millimetre", "dimension"="I/L", "is_si_unit"=TRUE, "category"="derived", "base_unit"="A/m", "conversion_reference"="DERIVED", "is_exact"=TRUE, "a"=0.0, "b"=1000.0, "c"=1.0, "d"=0.0, "underlying_def"="", "description"=""}, {"symbol"="A/m", "name"="ampere per metre", "dimension"="I/L", "is_si_unit"=TRUE, "category"="derived", "base_unit"="", "conversion_reference"="", "is_exact"=FALSE, "a"=0.0, "b"=0.0, "c"=0.0, "d"=0.0, "underlying_def"="", "description"=""}, {"symbol"="A/cm2", "name"="ampere per square centimetre", "dimension"="I/L2", "is_si_unit"=TRUE, "category"="derived", "base_unit"="A/m2", "conversion_reference"="DERIVED", "is_exact"=TRUE, "a"=0.0, "b"=10000.0, "c"=1.0, "d"=0.0, "underlying_def"="", "description"=""}, {"symbol"="A/ft2", "name"="ampere per square foot", "dimension"="I/L2", "is_si_unit"=TRUE, "category"="derived", "base_unit"="A/m2", "conversion_reference"="DERIVED", "is_exact"=TRUE, "a"=0.0, "b"=1.0, "c"=0.09290304, "d"=0.0, "underlying_def"="", "description"=""}, {"symbol"="A/mm2", "name"="ampere per square millimetre", "dimension"="I/L2", "is_si_unit"=TRUE, "category"="derived", "base_unit"="A/m2", "conversion_reference"="DERIVED", "is_exact"=TRUE, "a"=0.0, "b"=1000000.0, "c"=1.0, "d"=0.0, "underlying_def"="", "description"=""}, {"symbol"="mA/cm2", "name"="milliampere per square centimetre", "dimension"="I/L2", "is_si_unit"=TRUE, "category"="derived", "base_unit"="A/m2", "conversion_reference"="DERIVED", "is_exact"=TRUE, "a"=0.0, "b"=10.0, "c"=1.0, "d"=0.0, "underlying_def"="", "description"=""}, {"symbol"="mA/ft2", "name"="milliampere per square foot", "dimension"="I/L2", "is_si_unit"=TRUE, "category"="derived", "base_unit"="A/m2", "conversion_reference"="DERIVED", "is_exact"=TRUE, "a"=0.0, "b"=0.001, "c"=0.09290304, "d"=0.0, "underlying_def"="", "description"=""}, {"symbol"="uA/cm2", "name"="microampere per square centimetre", "dimension"="I/L2", "is_si_unit"=TRUE, "category"="derived", "base_unit"="A/m2", "conversion_reference"="DERIVED", "is_exact"=TRUE, "a"=0.0, "b"=0.01, "c"=1.0, "d"=0.0, "underlying_def"="", "description"=""}, {"symbol"="uA/in2", "name"="microampere per square inch", "dimension"="I/L2", "is_si_unit"=TRUE, "category"="derived", "base_unit"="A/m2", "conversion_reference"="DERIVED", "is_exact"=TRUE, "a"=0.0, "b"=1e-06, "c"=0.00064516, "d"=0.0, "underlying_def"="", "description"=""}, {"symbol"="A/m2", "name"="ampere per square metre", "dimension"="I/L2", "is_si_unit"=TRUE, "category"="derived", "base_unit"="", "conversion_reference"="", "is_exact"=FALSE, "a"=0.0, "b"=0.0, "c"=0.0, "d"=0.0, "underlying_def"="", "description"=""}, {"symbol"="1/H", "name"="per henry", "dimension"="I2T2/L2M", "is_si_unit"=TRUE, "category"="derived", "base_unit"="", "conversion_reference"="", "is_exact"=FALSE, "a"=0.0, "b"=0.0, "c"=0.0, "d"=0.0, "underlying_def"="", "description"=""}, {"symbol"="S", "name"="siemens", "dimension"="I2T3/L2M", "is_si_unit"=TRUE, "category"="atom-special", "base_unit"="", "conversion_reference"="", "is_exact"=FALSE, "a"=0.0, "b"=0.0, "c"=0.0, "d"=0.0, "underlying_def"="A/V", "description"="The electric conductance of a conductor in which a current of 1 A is produced by an electric \n\t\t\t\tpotential difference of 1 V. \n\t\t\t\tAlso known as a mho.\n\t\t\t"}, {"symbol"="cS", "name"="centisiemens", "dimension"="I2T3/L2M", "is_si_unit"=TRUE, "category"="prefixed", "base_unit"="S", "conversion_reference"="DERIVED", "is_exact"=TRUE, "a"=0.0, "b"=0.01, "c"=1.0, "d"=0.0, "underlying_def"="", "description"=""}, {"symbol"="dS", "name"="decisiemens", "dimension"="I2T3/L2M", "is_si_unit"=TRUE, "category"="prefixed", "base_unit"="S", "conversion_reference"="DERIVED", "is_exact"=TRUE, "a"=0.0, "b"=0.1, "c"=1.0, "d"=0.0, "underlying_def"="", "description"=""}, {"symbol"="ES", "name"="exasiemens", "dimension"="I2T3/L2M", "is_si_unit"=TRUE, "category"="prefixed", "base_unit"="S", "conversion_reference"="DERIVED", "is_exact"=TRUE, "a"=0.0, "b"=1e+18, "c"=1.0, "d"=0.0, "underlying_def"="", "description"=""}, {"symbol"="fS", "name"="femtosiemens", "dimension"="I2T3/L2M", "is_si_unit"=TRUE, "category"="prefixed", "base_unit"="S", "conversion_reference"="DERIVED", "is_exact"=TRUE, "a"=0.0, "b"=1e-15, "c"=1.0, 
